vi "Set Strings from Ref.vi"(8 "error in (no error)":errorcluster, 9 "Language Index (0)":i32, 10 "GObj Refnum":refnum<vi>, 11 "RingControl in":refnum<class "TabControl.lvclass">) -> (0 "error out":errorcluster, 3 "RingControl out":refnum<class "TabControl.lvclass">)   [LabVIEW 2013, in "SET Project Data.lvlib" / "TabControl.lvclass"]
uses:
  TabControl.lvclass
  Control/Control.lvclass
  SET Project Data.lvlib
  GObject/GObject.lvclass
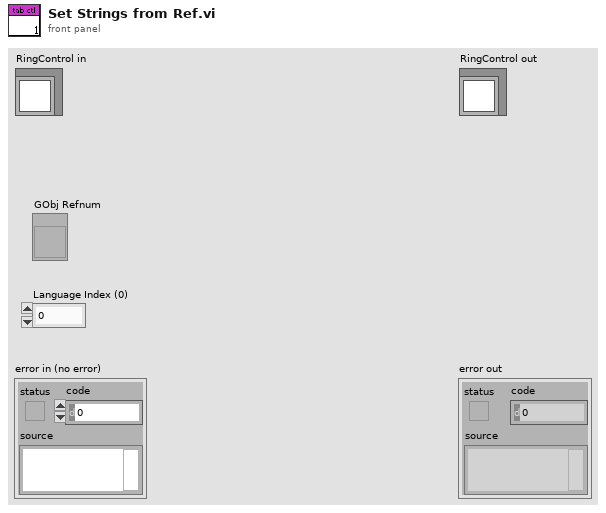
[diagram p1: front panel]
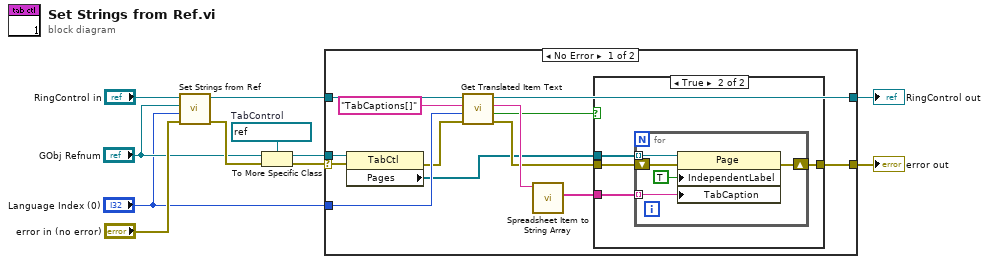
[diagram p0: block diagram]
diagram:
  w11 = refnum<vi> refnum  # TabControl
  n1 = call-parent "Set Strings from Ref.vi"("error in (no error)"="error in (no error)", "Language Index (0)"="Language Index (0)", "GObj Refnum"="GObj Refnum", "Control in"="RingControl in") -> ("error out"=w10:errorcluster, "Control out"=w7:refnum<class "TabControl.lvclass">)  [unwired: 6 in]
  n2 = To More Specific Class(target class=w11, reference="GObj Refnum", error in=w10) -> (specific class reference=w8:refnum<vi>, error out=w9:errorcluster)
  n3 = case shown="No Error" w9 {
    selector: w9 -> [w15 w35]
    tunnel: w8 -> [w14 _]
    tunnel: w7 -> [w23 w36]
    tunnel: "Language Index (0)" -> [w22 _]
    tunnel: [w21 w36] -> w2
    tunnel: [w16 w35] -> w1
    frame No Error {
      n4 = property class="TabCtl"(reference=w14, error in=w15) -> (error out=w13:errorcluster, "Pages"=w12:refnum<vi>[])  [unwired: 1 out]
      n5 = call "Get Translated Item Text.vi"("error in (no error)"=w13, "LangIndex (0)"=w22, "ItemName"="TabCaptions[]", "GObject in"=w23) -> ("error out"=w17:errorcluster, "Found?"=w19:bool, "Translated Text (ASCII)"=w20:string, "GObject out"=w21:refnum<class "TabControl.lvclass">)  [unwired: 4 in]
      n6 = call "Spreadsheet Item to String Array.vi"("Spreadsheet Item (ASCII)"=w20) -> ("Strings [] (ASCII)"=w18:string[])  [unwired: 10 in]
      n7 = case shown="True" w19 {
        tunnel: w18 -> [_ w29]
        tunnel: w17 -> [w25 w28]
        tunnel: [w25 w27] -> w16
        tunnel: w12 -> [_ w26]
        frame False {
        }
        frame True {
          n8 = for {
            tunnel: w29 -> [w31] mode=indexing
            tunnel: w26 -> [w32] mode=indexing
            shift-right: [w33] -> w27
            shift-left: w28 -> [w34]
            n9 = property class="Page"(reference=w32, error in=w34, "IndependentLabel"=TRUE ("Independent Label"), "TabCaption"=w31) -> (error out=w33:errorcluster)  [unwired: 1 out]
          }
        }
      }
    }
    frame Error {
    }
  }
  "error out" <- w1
  "RingControl out" <- w2
